vi "Read Boolean.vi"(7 "key":string, 8 "error in (no error)":errorcluster, 9 "default value":bool, 11 "Configuration File In":refnum<class "Configuration File.lvclass">) -> (0 "error out":errorcluster, 1 "value":bool, 3 "Configuration File Out":refnum<class "Configuration File.lvclass">)   [LabVIEW 2020, in "Configuration File.lvclass"]
doc: "High-level function for reading configuration file data from process class. If the specified key is not present, it is added with the configured default value."
uses:
  Configuration File.lvclass
  C:/Git/astemes-triarc-framework/source/Framework/Configuration/Configuration.lvclass
  Base/Base.lvclass/Base.ctl
  Base/Public/Read Base Name.vi
  Private/Read Config File Ref.vi
  Configuration/Protected/Get Config Ref.vi
  <vilib>/Utility/error.llb/Clear Errors.vi
  Process/Public/Read Name.vi
  <vilib>/Utility/config.llb/Not A Config Data Refnum.vi
  <vilib>/Utility/config.llb/Read Key (Boolean).vi
  Process/Process.lvclass
  Base/Base.lvclass
  <vilib>/Utility/config.llb/NI_LVConfig.lvlib
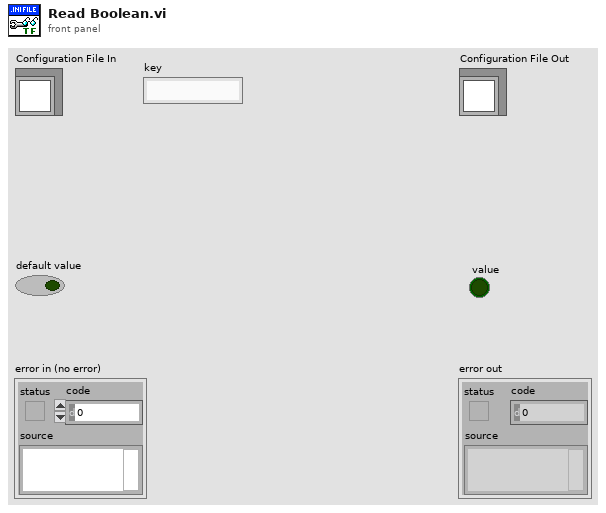
[diagram p1: front panel]
types:
  T1 = typedef "NI_LVConfig.lvlib/Config Data RefNum.ctl" = refnum<k1>
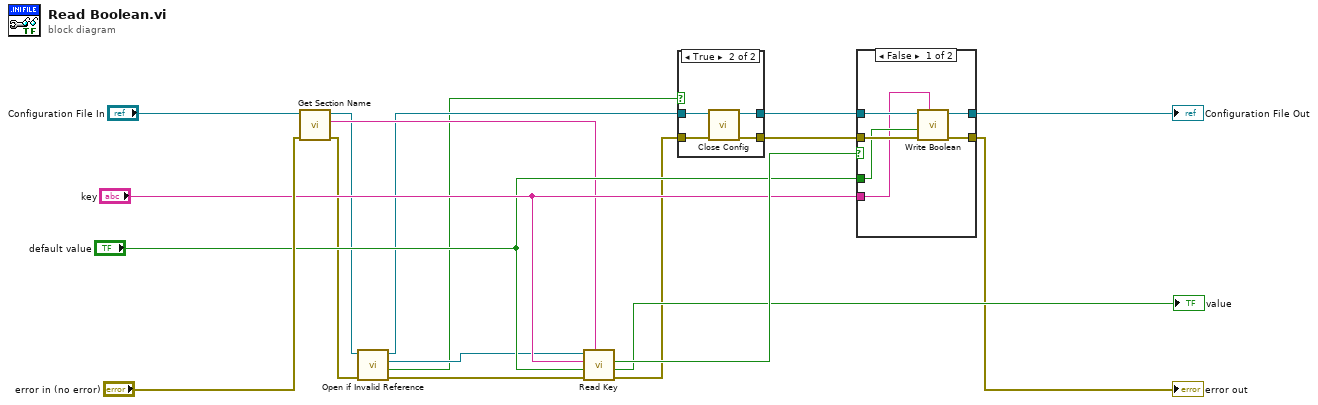
[diagram p0: block diagram]
diagram:
  n1 = call "Get Section Name.vi"("error in (no error)"="error in (no error)", "Configuration File In"="Configuration File In") -> ("error out"=w11:errorcluster, "Section Name"=w13:string, "Configuration File Out"=w10:refnum<class "Configuration File.lvclass">)  [unwired: 7 in]
  n2 = call "Open if Invalid Reference.vi"("error in (no error)"=w11, "Configuration File In"=w10) -> ("error out"=w9:errorcluster, "File opened?"=w1:bool, "refnum out"=w8:T1, "Configuration File Out"=w3:refnum<class "Configuration File.lvclass">)  [unwired: 6 in]
  n3 = call-poly <vilib>:"Read Key.vi"("section"=w13, "error in (no error)"=w9, "default value"="default value", "key"="key", "refnum"=w8) -> ("error out"=w6:errorcluster, "value"=→"value":bool, "found?"=w16:bool)  [unwired: 3 in, 1 out]
  n4 = case shown="True" w1 {
    tunnel: w6 -> [w19 w24]
    tunnel: [w19 w23] -> w4
    tunnel: w3 -> [w20 w22]
    tunnel: [w20 w21] -> w2
    frame False {
    }
    frame True {
      n5 = call-dynamic "Close Config.vi"("error in (no error)"=w24, "Configuration File File In"=w22) -> ("error out"=w23:errorcluster, "Configuration File File Out"=w21:refnum<class "Configuration File.lvclass">)  [unwired: 8 in]
    }
  }
  n6 = case shown="False" w16 {
    tunnel: w4 -> [w30 w32]
    tunnel: [w29 w32] -> w5
    tunnel: "key" -> [w25 _]
    tunnel: "default value" -> [w28 _]
    tunnel: w2 -> [w27 w31]
    tunnel: [w26 w31] -> w7
    frame False {
      n7 = call-dynamic "Write Boolean.vi"("key"=w25, "error in (no error)"=w30, "Value"=w28, "Configuration File In"=w27) -> ("error out"=w29:errorcluster, "Configuration File Out"=w26:refnum<class "Configuration File.lvclass">)  [unwired: 6 in]
    }
    frame True {
    }
  }
  "error out" <- w5
  "Configuration File Out" <- w7
